vi "Handle Dirty Fields for a Connection.vi"(9 "Field IDs":T1[](array[typedef])) -> (2 "String out":string)   [LabVIEW 2017]
uses:
  <vilib>/Rock Robotics/Network Tables/Field ID.ctl
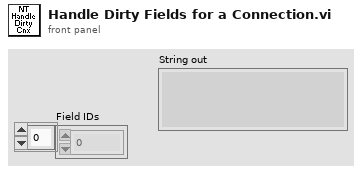
[diagram p1: front panel]
types:
  T1 = typedef "Field ID.ctl" = i32
  T2 = typedef "Field Data.ctl" = cluster{"Dbl":dbl, "String":string, "Type":T3, "Boolean":bool, "Sequence #":T4, "Flags":u8}
  T3 = typedef "Field Type.ctl" = enum8{"Invalid", "Bool", "Numeric", "String", "Raw", "Boolean Array", "Numeric Array", "String Array", "RPC"}
  T4 = typedef "Sequence.ctl" = u16
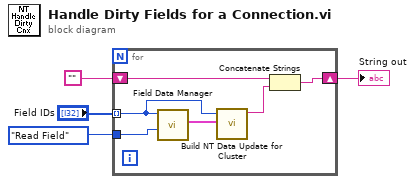
[diagram p0: block diagram]
diagram:
  n1 = for {
    tunnel: enum16{"Update Field", "Read Field"}."Read Field" ("Operation") -> [w10]
    tunnel: "Field IDs" -> [w5] mode=indexing
    shift-right: [w8] -> w4
    shift-left: "" -> [w7]
    n2 = call <vilib>:"Field Data Manager.vi"("Operation"=w10, "Field ID"=w5) -> ("Field Value Out"=w9:T2)  [unwired: 8 in, 1 out]
    n3 = call <vilib>:"Build NT Data Update for Cluster.vi"("Field Value"=w9, "Field ID"=w5) -> ("Data Buffer"=w6:string)  [unwired: 9 in]
    n4 = Concatenate Strings(w7, w6) -> (w8:string)
  }
  "String out" <- w4
